vi "侧铆试验判定.vi"(7 "Result":refnum<vi>, 10 "判定参数":T1, 11 "XY曲线":cluster{"X":dbl[], "Y":dbl[]}[](array[cluster])) -> (2 "判定项长度":i32, 3 "OK？":bool)   [LabVIEW 2020]
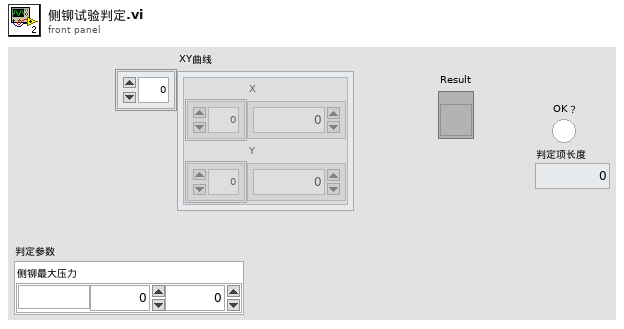
[diagram p1: front panel]
types:
  T1 = cluster{"侧铆最大压力":cluster{"单位":string, "下限":dbl, "上限":dbl}}
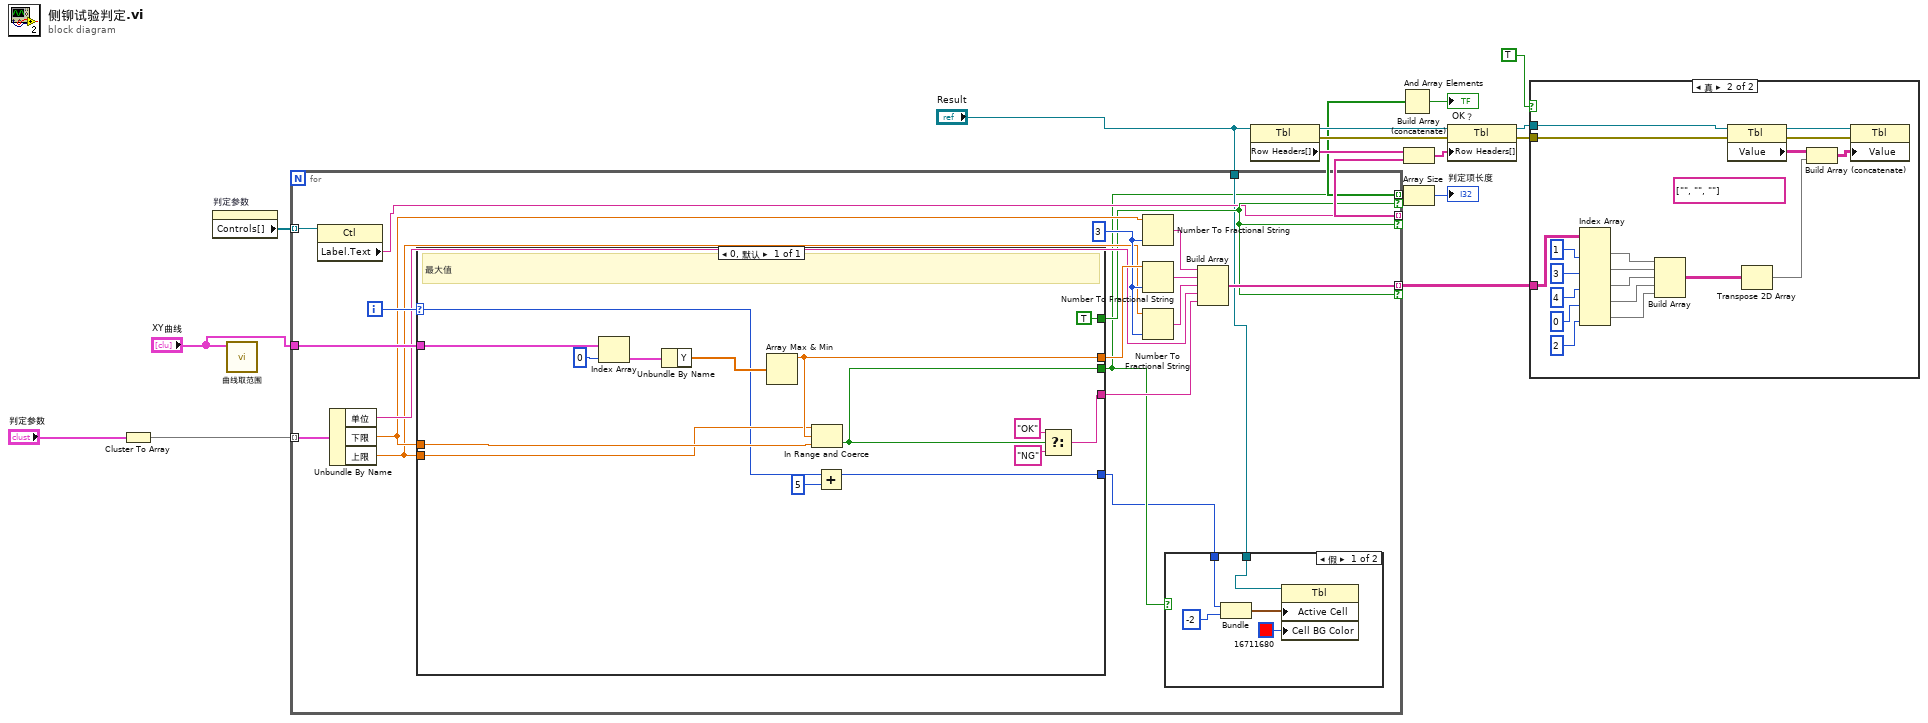
[diagram p0: block diagram]
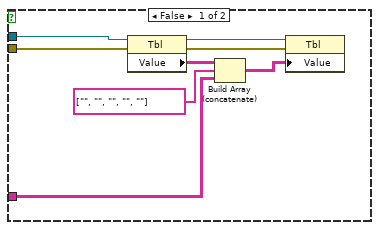
[diagram p2: hidden frame]
diagram:
  n1 = Cluster To Array(cluster="判定参数") -> (array=w17:cluster{"单位":string, "下限":dbl, "上限":dbl}[])
  n2 = property on="判定参数" class="Clust (严格)"() -> ("Controls[]"=w7:refnum<vi>[])  [unwired: 2 in, 2 out]
  n3 = call "曲线取范围.vi"("曲线In"="XY曲线") -> ()  [unwired: 10 in, 1 out]
  n4 = for {
    tunnel: w17 -> [w36] mode=indexing
    tunnel: w7 -> [w34] mode=indexing
    tunnel: "XY曲线" -> [w32]
    tunnel: [w19] -> w5 mode=indexing if=w22
    tunnel: [w23] -> w8 mode=indexing if=w22
    tunnel: [w21] -> w10 mode=indexing if=w22
    tunnel: "Result" -> [w20]
    i -> [w35]
    w31 = i16 3 ("精度(6)")
    n5 = property class="Ctl"(reference=w34) -> ("Label.Text"=w21:string)  [unwired: 1 in, 2 out]
    n6 = Unbundle By Name(w36) -> ("单位"=w26:string, "下限"=w25:dbl, "上限"=w24:dbl)
    n7 = case shown="0, 默认" w35 {
      selector: w35 -> [w44]
      tunnel: [w53] -> w33
      tunnel: w32 -> [w56]
      tunnel: [w50] -> w27
      tunnel: [w49] -> w19
      tunnel: w25 -> [w48]
      tunnel: w24 -> [w47]
      tunnel: [TRUE] -> w22
      tunnel: [w43] -> w18
      frame 0, Default {
        # "最大值"
        n8 = Index Array(array=w56, index=0 ("索引")) -> (element=w54:cluster{"X":dbl[], "Y":dbl[]})
        n9 = Unbundle By Name(w54) -> ("Y"=w45:dbl[])
        n10 = Array Max & Min(array=w45) -> (max value=w53:dbl)  [unwired: 3 out]
        n11 = In Range and Coerce(upper limit=w47, x=w53, lower limit=w48) -> (In Range?=w49:bool)  [unwired: 1 out]
        n12 = Add(x=w44, y=5) -> (x+y=w43:i32)
        n13 = Select(t="OK", s=w49, f="NG") -> (s? t:f=w50:string)
      }
    }
    n14 = Number To Fractional String(number=w25, precision (6)=w31) -> (F-format string=w30:string)  [unwired: 2 in]
    n15 = Number To Fractional String(number=w33, precision (6)=w31) -> (F-format string=w29:string)  [unwired: 2 in]
    n16 = Number To Fractional String(number=w24, precision (6)=w31) -> (F-format string=w28:string)  [unwired: 2 in]
    n17 = case shown="假" w19 {
      tunnel: w20 -> [w41 _]
      tunnel: w18 -> [w37 _]
      frame False {
        n18 = Bundle(w37, "索引"=-2) -> (w38:cluster{i32, "索引":i32})  [unwired: 1 in]
        n19 = property class="Tbl"(reference=w41, "Active Cell"=w38, "Cell BG Color"=u32 16711680 ("活动单元格:单元格背景色")) -> ()  [unwired: 1 in, 2 out]
      }
      frame True {
      }
    }
    n20 = Build Array(w30, w29, w28, w26, w27) -> (w23:string[])
  }
  n21 = property class="Tbl"(reference="Result") -> (reference out=w12:refnum<vi>, error out=w15:errorcluster, "Row Headers[]"=w9:string[])  [unwired: 1 in]
  n22 = And Array Elements(Boolean array=w5) -> (logical AND=→"OK？":bool)
  n23 = Build Array (concatenate)(w9, w10) -> (w11:string[])
  n24 = Array Size(array=w5) -> (size(s)=→"判定项长度":i32)
  n25 = property class="Tbl"(reference=w12, error in=w15, "Row Headers[]"=w11) -> (reference out=w13:refnum<vi>, error out=w14:errorcluster)
  n26 = case shown="真" TRUE {
    tunnel: w14 -> [w62 w81]
    tunnel: w13 -> [w59 w78]
    tunnel: w8 -> [w58 w70]
    frame False {
      n27 = property class="Tbl"(reference=w59, error in=w62) -> (reference out=w60:refnum<vi>, error out=w61:errorcluster, "Value"=w63:string[][])
      n28 = Build Array (concatenate)(w63, string[] ["", "", "", "", ""], w58) -> (w64:string[][])
      n29 = property class="Tbl"(reference=w60, error in=w61, "Value"=w64) -> ()  [unwired: 2 out]
    }
    frame True {
      (unwired) string[] ["", "", ""]
      n30 = Index Array(array=w70, index (col) #1=1 ("禁用的索引 (列)"), index (col) #2=3 ("索引 (列)"), index (col) #3=4 ("索引 (列)"), index (col) #4=0 ("索引 (列)"), index (col) #5=2 ("索引 (列)")) -> (element #1=w74:string[], element #2=w75:string[], element #3=w76:string[], element #4=w66:string[], element #5=w65:string[])  [unwired: 5 in]
      n31 = Build Array(w74, w75, w76, w66, w65) -> (w77:string[][])
      n32 = property class="Tbl"(reference=w78, error in=w81) -> (reference out=w79:refnum<vi>, error out=w80:errorcluster, "Value"=w82:string[][])
      n33 = Transpose 2D Array(2D array=w77) -> (transposed array=w69:string[][])
      n34 = Build Array (concatenate)(w82, w69) -> (w83:string[][])
      n35 = property class="Tbl"(reference=w79, error in=w80, "Value"=w83) -> ()  [unwired: 2 out]
    }
  }
